vi "PhidgetRemoveServer.vi"(8 "error in":errorcluster, 10 "flags":i32, 11 "name":string) -> (0 "error out":errorcluster)   [LabVIEW 2012, in "Phidget Common.lvlib"]
doc: "${RemoveServer:Header}"
uses:
  <instrlib>/Phidgets/Phidget Common/Phidget Common.lvlib
  phidget22.dll
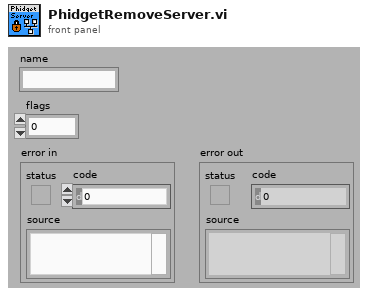
[diagram p1: front panel]
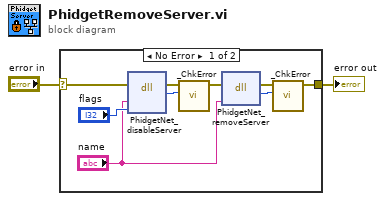
[diagram p0: block diagram]
diagram:
  n1 = case shown="No Error" "error in" {
    selector: "error in" -> [w6 w12]
    tunnel: [w9 w12] -> w1
    frame No Error {
      n2 = dll-call lib="phidget22.dll" fn="PhidgetNet_disableServer"(error in=w6, "name"="name", "flags"="flags") -> (error out=w5:errorcluster, "return type"=w3:i32)  [unwired: 4 in, 1 out]
      n3 = call <instrlib>:"_ChkError.vi"("Return Code"=w3, "error in (no error)"=w5) -> ("error out"=w4:errorcluster)  [unwired: 9 in]
      n4 = dll-call lib="phidget22.dll" fn="PhidgetNet_removeServer"(error in=w4, "name"="name") -> (error out=w10:errorcluster, "return type"=w11:i32)  [unwired: 3 in, 1 out]
      n5 = call <instrlib>:"_ChkError.vi"("Return Code"=w11, "error in (no error)"=w10) -> ("error out"=w9:errorcluster)  [unwired: 9 in]
    }
    frame Error {
    }
  }
  "error out" <- w1
